vi "Wait Multi With Memory.vi"(8 "error in (no error)":errorcluster, 9 "Timeout in ms (-1)":i32=-1, 10 "Ignore previous (F)":bool, 11 "Notifiers in":refnum<class "Notifier.lvclass">[](array[class])) -> (0 "error out":errorcluster, 1 "Timed out?":bool, 2 "Data Notifications":refnum<class "Data.lvclass">[](array[class]), 3 "Notifiers dub":refnum<class "Notifier.lvclass">[](array[class]))   [LabVIEW 2020, in "Data.lvlib" / "Notifier.lvclass"]
doc: "Wait on notification from multiple notifiers with notification history."
uses:
  Notifier.lvclass
  Data.lvclass
  Notifier.lvclass/Notifier.ctl
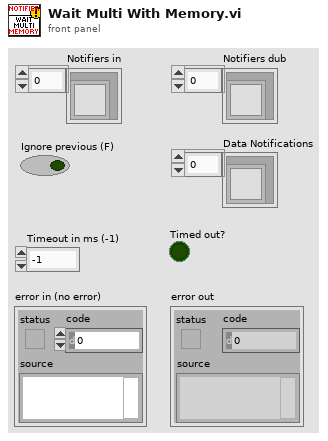
[diagram p1: front panel]
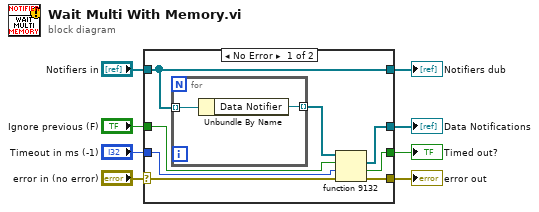
[diagram p0: block diagram]
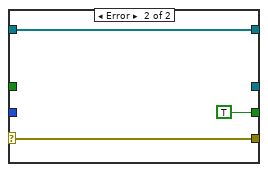
[diagram p2: hidden frame]
diagram:
  n1 = case shown="No Error" "error in (no error)" {
    selector: "error in (no error)" -> [w16 w21]
    tunnel: [w15 w21] -> w7
    tunnel: [w9 w20] -> w5
    tunnel: "Notifiers in" -> [w9 w20]
    tunnel: [w14 _] -> w4
    tunnel: "Timeout in ms (-1)" -> [w13 _]
    tunnel: "Ignore previous (F)" -> [w12 _]
    tunnel: [w11 TRUE ("timed out?")] -> w1
    frame No Error {
      n2 = for {
        tunnel: w9 -> [w18] mode=indexing
        tunnel: [w17] -> w10 mode=indexing
        n3 = Unbundle By Name(w18) -> ("Data Notifier"=w17:refnum<notifier>)
      }
      n4 = fn#9132(0:w10, 1:w12, 2:w13, 3:w16) -> (9:w14:refnum<class "Data.lvclass">[], 10:w11:bool, 11:w15:errorcluster)  [unwired: 1 out]
    }
    frame Error {
    }
  }
  "error out" <- w7
  "Notifiers dub" <- w5
  "Data Notifications" <- w4
  "Timed out?" <- w1
